vi "Chebeval.vi"(9 "degree":u16=2, 10 "Cheby weights":dbl[](array[numeric]), 11 "x":dbl[](array[numeric])) -> (3 "y":dbl[](array[numeric]))   [LabVIEW 2025]
panel:
  out "Array":dbl[][](array[numeric])
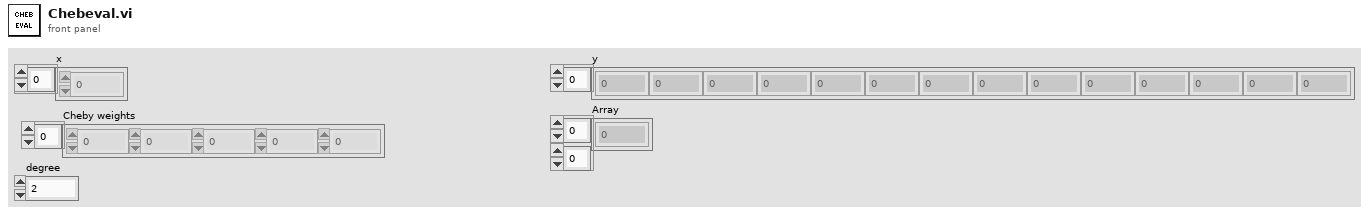
[diagram p1: front panel]
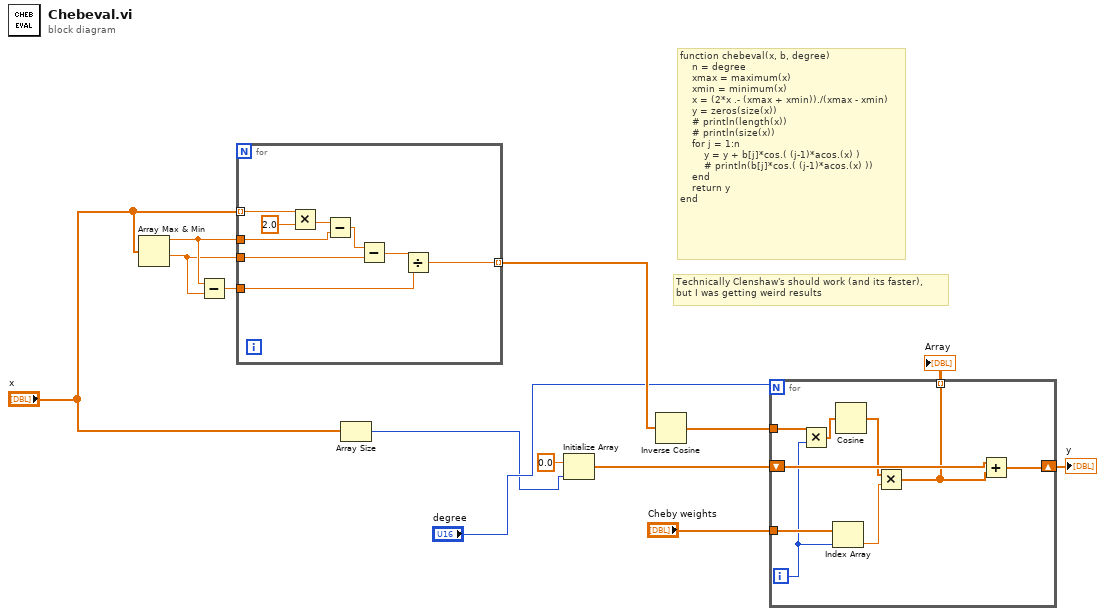
[diagram p0: block diagram]
diagram:
  # "Technically Clenshaw's should work (and its faster),\nbut I was getting weird results"
  # "function chebeval(x, b, degree)\n    n = degree\n    xmax = maximum(x)\n    xmin = minimum(x)\n    x = (2*x .- (xmax + xmin))./(xmax - xmin)\n    y = zeros(size(x))\n    # println(length(x))\n    # println(size(x))\n    for j = 1:n\n        y = y + b[j]*cos.( (j-1)*acos.(x) )\n        # println(b[j]*cos.( (j-1)*acos.(x) ))\n    end\n    return y\nend"
  n1 = Array Max & Min(array="x") -> (max value=w12:dbl, min value=w11:dbl)  [unwired: 2 out]
  n2 = Subtract(x=w12, y=w11) -> (x-y=w10:dbl)
  n3 = for {
    tunnel: "x" -> [w22] mode=indexing
    tunnel: w12 -> [w19]
    tunnel: w11 -> [w17]
    tunnel: w10 -> [w15]
    tunnel: [w14] -> w6 mode=indexing
    n4 = Multiply(x=w22, y=2.0) -> (x*y=w20:dbl)
    n5 = Subtract(x=w20, y=w19) -> (x-y=w18:dbl)
    n6 = Subtract(x=w18, y=w17) -> (x-y=w16:dbl)
    n7 = Divide(x=w16, y=w15) -> (x/y=w14:dbl)
  }
  n8 = Array Size(array="x") -> (size(s)=w1:i32)
  n9 = Initialize Array(0.0 ("element"), w1) -> (w9:dbl[])
  n10 = Inverse Cosine(1:w6) -> (0:w8:dbl[])
  n11 = for {
    N: "degree" -> [_]
    shift-right: [w27] -> w5
    shift-left: w9 -> [w28]
    tunnel: w8 -> [w31]
    tunnel: "Cheby weights" -> [w30]
    tunnel: [w26] -> w4 mode=indexing
    i -> [w23]
    n12 = Multiply(x=w31, y=w23) -> (x*y=w25:dbl[])
    n13 = Index Array(array=w30, index=w23) -> (element=w29:dbl)
    n14 = Cosine(x=w25) -> (cos(x)=w24:dbl[])
    n15 = Multiply(x=w24, y=w29) -> (x*y=w26:dbl[])
    n16 = Add(x=w28, y=w26) -> (x+y=w27:dbl[])
  }
  "y" <- w5
  "Array" <- w4
